vi "Write.vi"(0 "wait for ack (F)":bool, 1 "timeout in ms (-1)":i32=-1, 5 "element":T1, 7 "element valid? (T)":bool=TRUE, 9 "last element? (F)":bool, 11 "subchannel (0)":i32, 12 "size (unlimited)":i32) -> (3 "timed out?":bool, 4 "count":i32, 6 "channel":T2, 10 "id":u32)   [LabVIEW 2019, in "MessengerM.lvlib"]
doc: "Writes an element to a Messenger channel. The endpoint waits if the channel is full."
uses:
  <resource>/Channels/MessengerM/MessengerM.lvlib
  <resource>/Channels/MessengerM/))Channel.ctl
  <resource>/Channels/MessengerM/Element.ctl
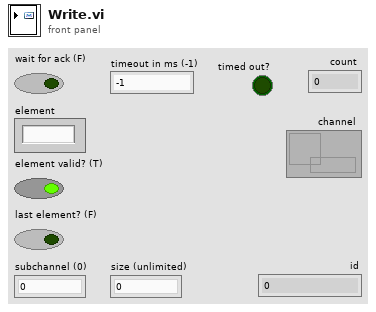
[diagram p1: front panel]
types:
  T1 = typedef "MessengerM.lvlib/Element.ctl" = string
  T2 = typedef "MessengerM.lvlib/))Channel.ctl" = refnum<queue>
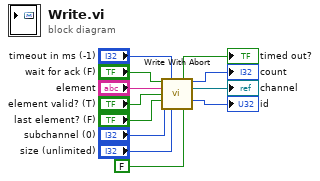
[diagram p0: block diagram]
diagram:
  n1 = call <resource>:"Write With Abort.vi"("wait for ack (F)"="wait for ack (F)", "timeout in ms (-1)"="timeout in ms (-1)", "element"="element", "element valid? (T)"="element valid? (T)", "last element? (F)"="last element? (F)", "subchannel (0)"="subchannel (0)", "size (unlimited)"="size (unlimited)", "abort (F)"=FALSE) -> ("timed out?"=→"timed out?":bool, "count"=→"count":i32, "channel"=→"channel":T2, "id"=→"id":u32)  [unwired: 3 in, 1 out]
